vi "bonsai point grey workflow example.vi"() -> ()   [LabVIEW 2010]
panel:
  in  "Copy 2":bool
  in  "exit":bool
  out "Notes":string="The suggestion is to use this workflow in order to save the necessary Metadata from the camera. The metadata are created on the camera's hardware, which means that the software delays/lags are not present."
  # "Bonsai workflow to save PointGrey metadata (FrameCounter\nand TimeStamp), essential for correct alignment with data."
  # "Then, execute Ctrl+V on Bonsai's Workflow to paste it.\nChange the FileName on the CsvWriter according to your needs."
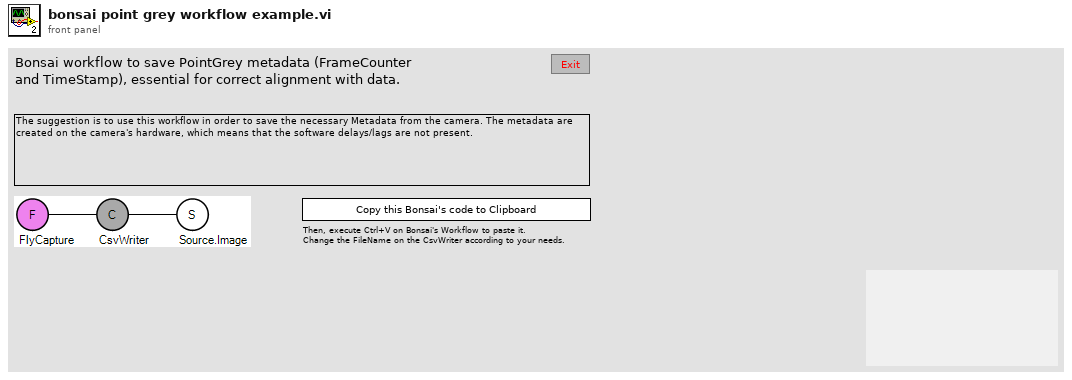
[diagram p1: front panel]
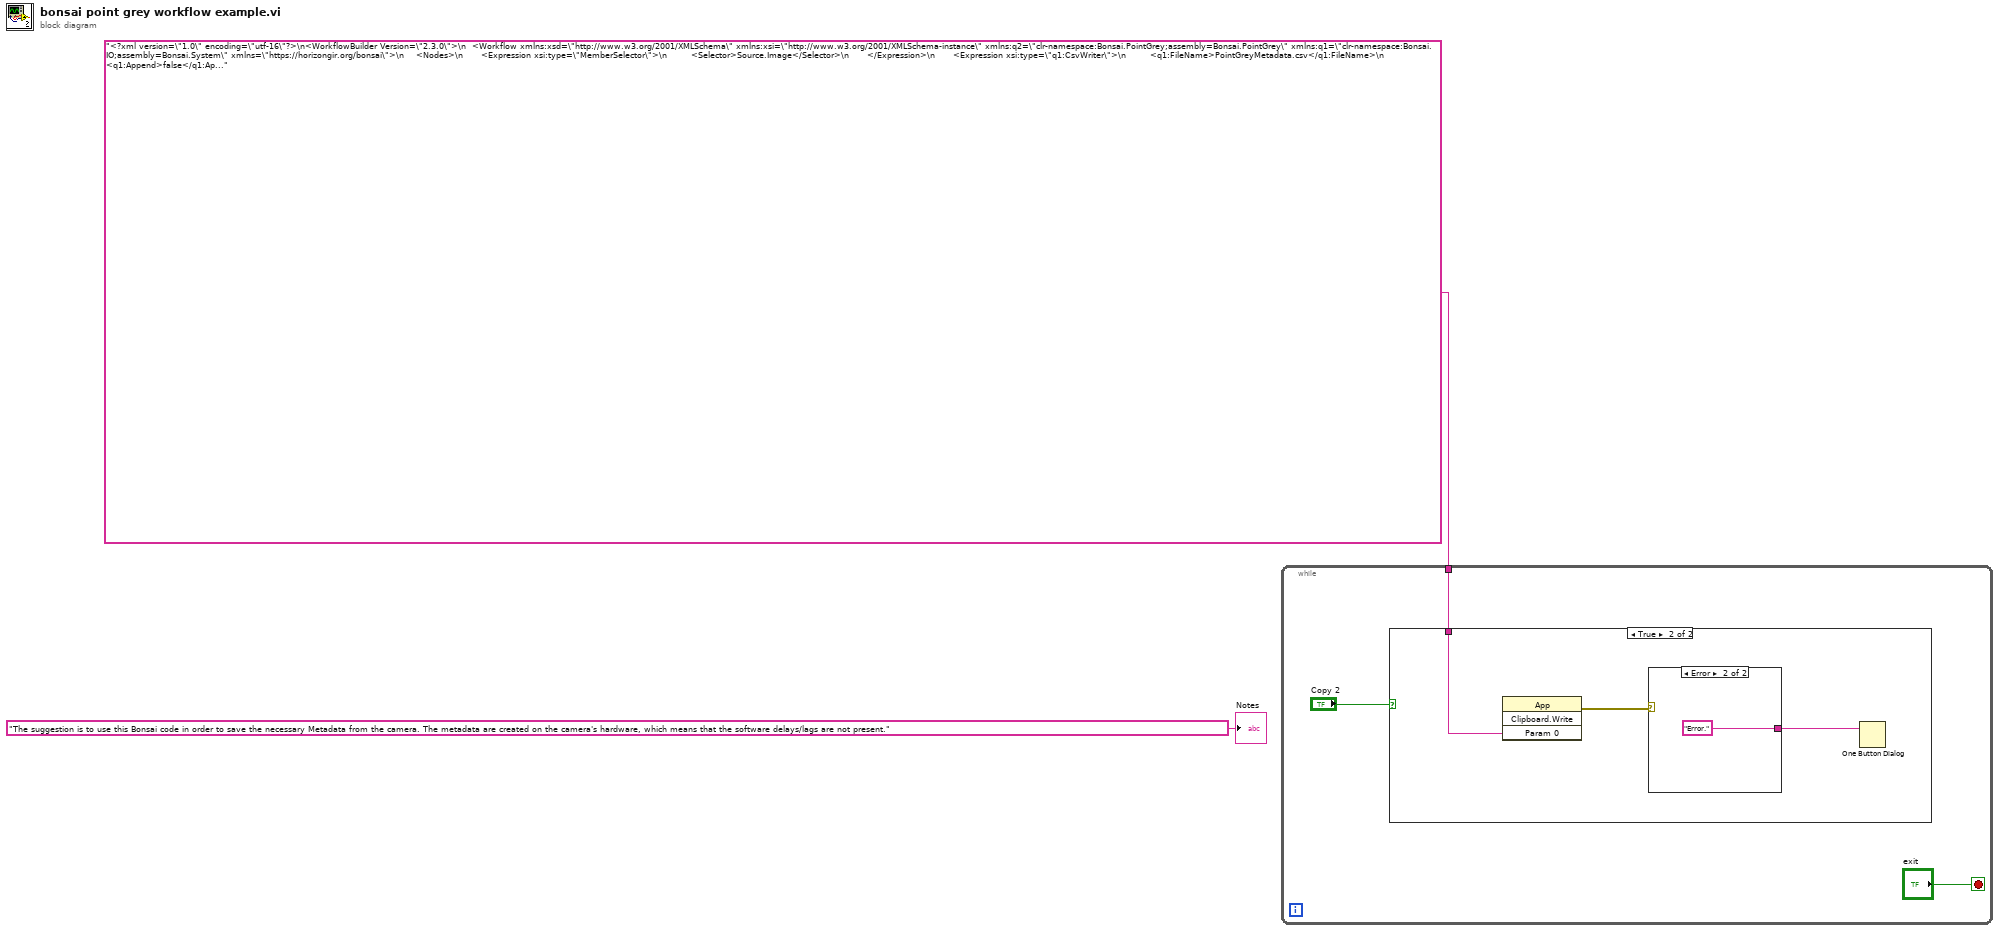
[diagram p0: block diagram]
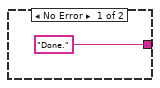
[diagram p3: hidden frame]
diagram:
  n1 = while {
    tunnel: "<?xml version=\"1.0\" encoding=\"utf-16\"?>\n<WorkflowBuilder Version=\"2.3.0\">\n  <Workflow xmlns:xsd=\"http://www.w3.org/2001/XMLSchema\" xmlns:xsi=\"http://www.w3.org/2001/XMLSchema-instance\" xmlns:q2=\"clr-namespace:Bonsai.PointGrey;assembly=Bonsai.PointGrey\" xmlns:q1=\"clr-namespace:Bonsai.IO;assembly=Bonsai.System\" xmlns=\"https://horizongir.org/bonsai\">\n    <Nodes>\n      <Expression xsi:type=\"MemberSelector\">\n        <Selector>Source.Image</Selector>\n      </Expression>\n      <Expression xsi:type=\"q1:CsvWriter\">\n        <q1:FileName>PointGreyMetadata.csv</q1:FileName>\n        <q1:Append>false</q1:Append>\n        <q1:Overwrite>false</q1:Overwrite>\n        <q1:Suffix>Timestamp</q1:Suffix>\n        <q1:IncludeHeader>false</q1:IncludeHeader>\n        <q1:Selector>Source.Metadata.embeddedFrameCounter,Source.Metadata.embeddedTimeStamp</q1:Selector>\n      </Expression>\n      <Expression xsi:type=\"Combinator\">\n        <Combinator xsi:type=\"q2:FlyCapture\">\n          <q2:Index>0</q2:Index>\n          <q2:ColorProcessing>Default</q2:ColorProcessing>\n        </Combinator>\n      </Expression>\n    </Nodes>\n    <Edges>\n      <Edge>\n        <From>1</From>\n        <To>0</To>\n        <Label>Source1</Label>\n      </Edge>\n      <Edge>\n        <From>2</From>\n        <To>1</To>\n        <Label>Source1</Label>\n      </Edge>\n    </Edges>\n  </Workflow>\n  <ExtensionTypes>\n    <Type>Bonsai.IO.CsvWriter, Bonsai.System, Version=2.3.0.0, Culture=neutral, PublicKeyToken=null</Type>\n    <Type>Bonsai.PointGrey.FlyCapture, Bonsai.PointGrey, Version=2.3.0.0, Culture=neutral, PublicKeyToken=null</Type>\n  </ExtensionTypes>\n</WorkflowBuilder>" ("message") -> [w3]
    stop <- "exit" stop-if-true
    n2 = case shown="True" "Copy 2" {
      tunnel: w3 -> [_ w6]
      frame False {
      }
      frame True {
        n3 = invoke class="App" method="Clipboard.Write"("Param 0"=w6) -> (error out=w8:errorcluster)  [unwired: 3 in, 3 out]
        n4 = case shown="Error" w8 {
          tunnel: ["Done." ("message") "Error." ("message")] -> w7
          frame No Error {
          }
          frame Error {
          }
        }
        n5 = One Button Dialog(message=w7) -> ()  [unwired: 1 in, 1 out]
      }
    }
  }
  "Notes" <- "The suggestion is to use this Bonsai code in order to save the necessary Metadata from the camera. The metadata are created on the camera's hardware, which means that the software delays/lags are not present." ("Notes")
